vi "CloseSensorSession.vi"(8 "error in (no error)":errorcluster, 11 "RoomAlert in":refnum<class "RoomAlert.lvclass">) -> (0 "error out":errorcluster, 3 "RoomAlert out":refnum<class "RoomAlert.lvclass">)   [LabVIEW 2018, in "SensorPlugins.lvlib" / "RoomAlert.lvclass"]
doc: "Closes the session to the instrument."
uses:
  RoomAlert.lvclass
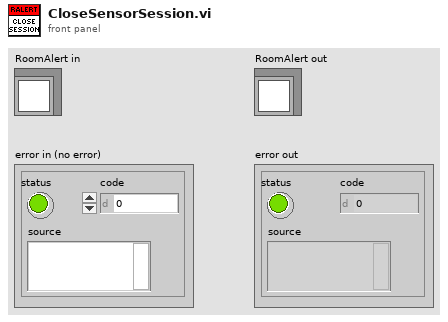
[diagram p1: front panel]
types:
  T1 = typedef "SensorPlugins.lvlib/RoomAlert.lvclass/RoomAlertControls.ctl" = cluster{"Connected?":bool, "IP Address of SNMP Device":string, "Port (161)":u16, "Community Name":string, "Measurements To Read Array":u16[], "Update LightTower?":bool, "LightTower":cluster{"Red":bool, "Amber":bool, "Green":bool, "Audio":bool}, "RoomAlert Model ID":string, "Sensor OID Numbers":string[][], "Sensor Light Tower OID Numbers":string[][]}[]
  T2 = typedef "SensorPlugins.lvlib/RoomAlert.lvclass/CommunicationControls.ctl" = refnum<k16>[]
  T3 = cluster{"Connected?":bool, "IP Address of SNMP Device":string, "Port (161)":u16, "Community Name":string, "Measurements To Read Array":u16[], "Update LightTower?":bool, "LightTower":cluster{"Red":bool, "Amber":bool, "Green":bool, "Audio":bool}, "RoomAlert Model ID":string, "Sensor OID Numbers":string[][], "Sensor Light Tower OID Numbers":string[][]}
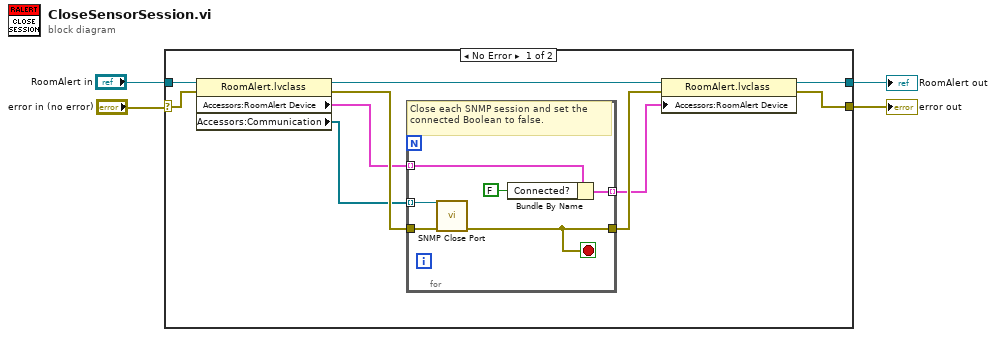
[diagram p0: block diagram]
diagram:
  n1 = case shown="No Error" "error in (no error)" {
    selector: "error in (no error)" -> [w13 w21]
    tunnel: "RoomAlert in" -> [w14 w22]
    tunnel: [w10 w22] -> w2
    tunnel: [w9 w21] -> w1
    frame No Error {
      n2 = property class="RoomAlert.lvclass"(reference=w14, error in=w13) -> (reference out=w11:refnum<class "RoomAlert.lvclass">, error out=w12:errorcluster, "Accessors:RoomAlert Device"=w7:T1, "Accessors:Communication "=w6:T2)
      n3 = for {
        tunnel: w12 -> [w17]
        tunnel: [w16] -> w8
        tunnel: w6 -> [w15] mode=indexing
        tunnel: w7 -> [w20] mode=indexing
        tunnel: [w18] -> w5 mode=indexing
        stop <- w16 stop-if-true
        # "Close each SNMP session and set the connected Boolean to false."
        n4 = call "SNMP Close Port.vi"("error in (no error)"=w17, "connection ID"=w15) -> ("error out"=w16:errorcluster)  [unwired: 9 out]
        n5 = Bundle By Name(cluster=w20, "Connected?"=FALSE) -> (w18:T3)
      }
      n6 = property class="RoomAlert.lvclass"(reference=w11, error in=w8, "Accessors:RoomAlert Device"=w5) -> (reference out=w10:refnum<class "RoomAlert.lvclass">, error out=w9:errorcluster)
    }
    frame Error {
    }
  }
  "error out" <- w1
  "RoomAlert out" <- w2
